vi "Day 5.2 - overlap with diagnals.vi"(11 "input":string[](array[string])) -> (3 "output":u32)   [LabVIEW 2021]
uses:
  Controls/Thermal position.ctl
  Controls/vent position.ctl
panel:
  out "Intensity Graph":i32[][](graph)
  out "vents":i32[][](array[numeric])
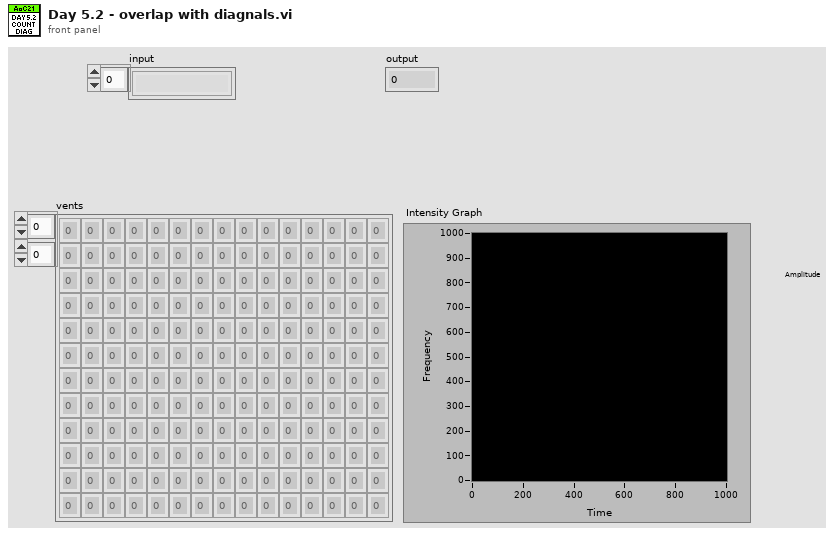
[diagram p1: front panel]
types:
  T1 = typedef "Thermal position.ctl" = cluster{"Start Vent position":T2, "End Vent position":T2}
  T2 = typedef "vent position.ctl" = cluster{"x":i32, "y":i32}
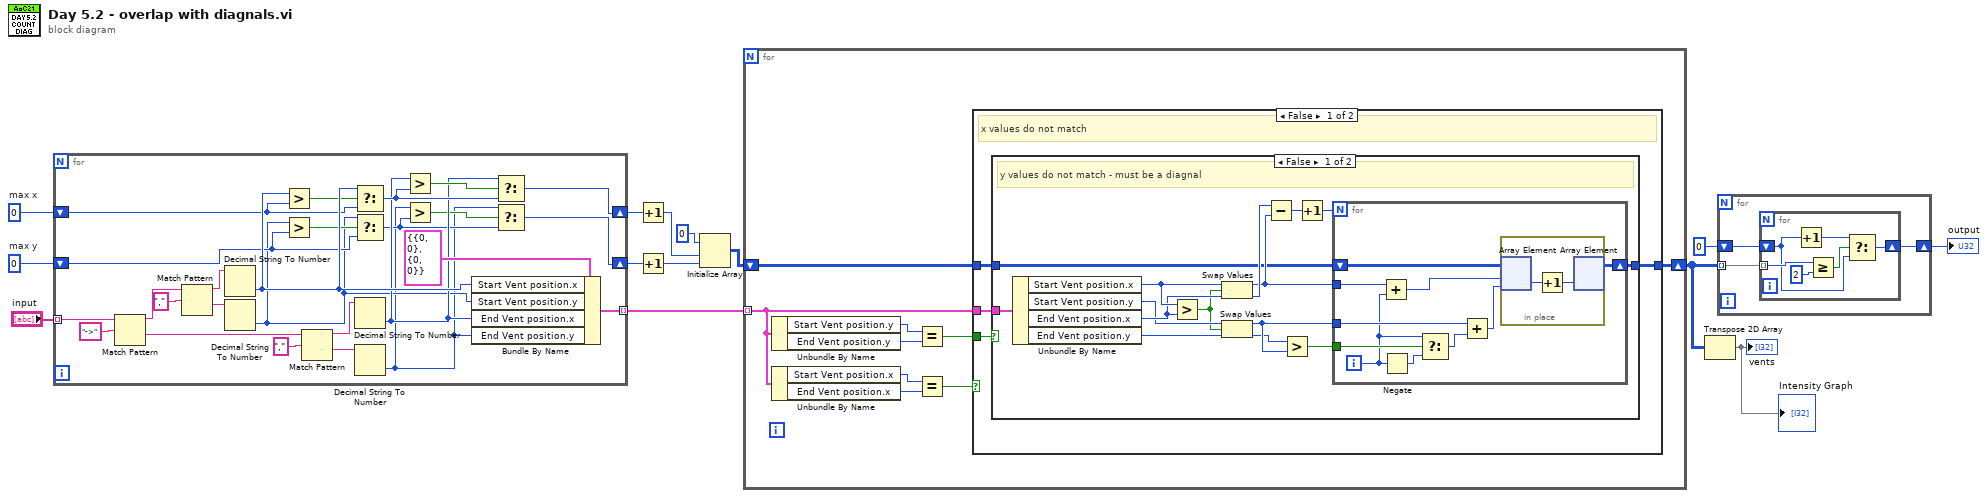
[diagram p0: block diagram]
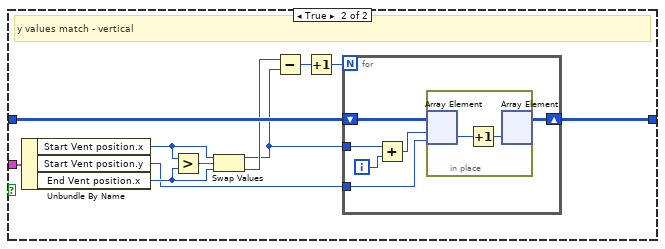
[diagram p2: hidden frame]
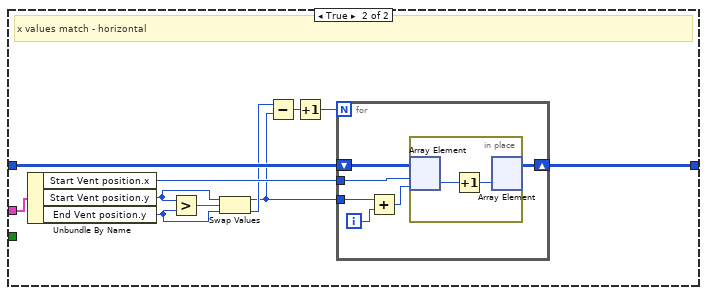
[diagram p3: hidden frame]
diagram:
  w11 = 0  # max y
  w12 = 0  # max x
  n1 = for {
    tunnel: "input" -> [w40] mode=indexing
    tunnel: [w29] -> w13 mode=indexing
    shift-right: [w24] -> w9
    shift-left: w12 -> [w26]
    shift-right: [w18] -> w8
    shift-left: w11 -> [w17]
    n2 = Match Pattern(string=w40, regular expression="->") -> (before substring=w38:string, after substring=w35:string)  [unwired: 1 in, 2 out]
    n3 = Match Pattern(string=w38, regular expression=",") -> (before substring=w32:string, after substring=w31:string)  [unwired: 1 in, 2 out]
    n4 = Decimal String To Number(string=w32) -> (number=w28:i32)  [unwired: 2 in, 1 out]
    n5 = Decimal String To Number(string=w31) -> (number=w16:i32)  [unwired: 2 in, 1 out]
    n6 = Greater?(x=w28, y=w26) -> (0:w27:bool)
    n7 = Greater?(x=w16, y=w17) -> (0:w21:bool)
    n8 = Match Pattern(string=w35, regular expression=",") -> (before substring=w34:string, after substring=w33:string)  [unwired: 1 in, 2 out]
    n9 = Select(t=w28, s=w27, f=w26) -> (s? t:f=w23:i32)
    n10 = Select(t=w16, s=w21, f=w17) -> (s? t:f=w19:i32)
    n11 = Decimal String To Number(string=w34) -> (number=w22:i32)  [unwired: 2 in, 1 out]
    n12 = Decimal String To Number(string=w33) -> (number=w15:i32)  [unwired: 2 in, 1 out]
    n13 = Greater?(x=w22, y=w23) -> (0:w25:bool)
    n14 = Greater?(x=w15, y=w19) -> (0:w20:bool)
    n15 = Bundle By Name(cluster=T1 {"Start Vent position"={"x"=0, "y"=0}, "End Vent position"={"x"=0, "y"=0}} ("Hydrothermal"), "Start Vent position.x"=w28, "Start Vent position.y"=w16, "End Vent position.x"=w22, "End Vent position.y"=w15) -> (w29:T1)
    n16 = Select(t=w22, s=w25, f=w23) -> (s? t:f=w24:i32)
    n17 = Select(t=w15, s=w20, f=w19) -> (s? t:f=w18:i32)
  }
  n18 = Increment(x=w9) -> (x+1=w6:i32)
  n19 = Increment(x=w8) -> (x+1=w5:i32)
  n20 = Initialize Array(0, w6, w5) -> (w7:i32[][])
  n21 = for {
    tunnel: w13 -> [w42] mode=indexing
    shift-right: [w41] -> w2
    shift-left: w7 -> [w44]
    n22 = Unbundle By Name(w42) -> ("Start Vent position.y"=w49:i32, "End Vent position.y"=w48:i32)
    n23 = Unbundle By Name(w42) -> ("Start Vent position.x"=w46:i32, "End Vent position.x"=w45:i32)
    n24 = Equal?(x=w49, y=w48) -> (x = y?=w43:bool)
    n25 = Equal?(x=w46, y=w45) -> (x = y?=w47:bool)
    n26 = case shown="False" w47 {
      tunnel: w44 -> [w51 w110]
      tunnel: [w50 w104] -> w41
      tunnel: w43 -> [w53 _]
      tunnel: w42 -> [w52 w101]
      frame False {
        # "x values do not match"
        n27 = case shown="False" w53 {
          tunnel: [w61 w88] -> w50
          tunnel: w52 -> [w60 w91]
          tunnel: w51 -> [w62 w87]
          frame False {
            # "y values do not match - must be a diagnal"
            n28 = Unbundle By Name(w60) -> ("Start Vent position.x"=w65:i32, "Start Vent position.y"=w59:i32, "End Vent position.x"=w64:i32, "End Vent position.y"=w58:i32)
            n29 = Greater?(x=w65, y=w64) -> (0:w57:bool)
            n30 = Swap Values(12:w65, 13:w57, 14:w64) -> (1:w66:i32, 3:w67:i32)
            n31 = Swap Values(12:w59, 13:w57, 14:w58) -> (1:w55:i32, 3:w54:i32)
            n32 = Subtract(x=w67, y=w66) -> (x-y=w68:i32)
            n33 = Greater?(x=w54, y=w55) -> (0:w56:bool)
            n34 = Increment(x=w68) -> (x+1=w63:i32)
            n35 = for {
              N: w63 -> [_]
              tunnel: w66 -> [w78]
              shift-right: [w75] -> w61
              shift-left: w62 -> [w77]
              tunnel: w55 -> [w74]
              tunnel: w56 -> [w72]
              i -> [w69]
              n36 = Add(x=w78, y=w69) -> (x+y=w76:i32)
              n37 = Negate(x=w69) -> (-x=w71:i32)
              n38 = Select(t=w69, s=w72, f=w71) -> (s? t:f=w70:i32)
              n39 = Add(x=w74, y=w70) -> (x+y=w73:i32)
              n40 = in-place {
                n41 = in-place-array #1(w77, w76, w73) -> (w80:i32)
                n42 = Increment(x=w80) -> (x+1=w79:i32)
                n43 = in-place-array #1(w79) -> (w75:i32[][])  [unwired: 2 out]
              }
            }
          }
          frame True {
            # "y values match - vertical"
            n44 = Unbundle By Name(w91) -> ("Start Vent position.x"=w84:i32, "Start Vent position.y"=w82:i32, "End Vent position.x"=w83:i32)
            n45 = Greater?(x=w84, y=w83) -> (0:w90:bool)
            n46 = Swap Values(12:w84, 13:w90, 14:w83) -> (1:w85:i32, 3:w86:i32)
            n47 = Subtract(x=w86, y=w85) -> (x-y=w89:i32)
            n48 = Increment(x=w89) -> (x+1=w81:i32)
            n49 = for {
              N: w81 -> [_]
              tunnel: w82 -> [w93]
              tunnel: w85 -> [w96]
              shift-right: [w92] -> w88
              shift-left: w87 -> [w95]
              i -> [w97]
              n50 = Add(x=w96, y=w97) -> (x+y=w94:i32)
              n51 = in-place {
                n52 = in-place-array #2(w95, w94, w93) -> (w99:i32)
                n53 = Increment(x=w99) -> (x+1=w98:i32)
                n54 = in-place-array #2(w98) -> (w92:i32[][])  [unwired: 2 out]
              }
            }
          }
        }
      }
      frame True {
        # "x values match - horizontal"
        n55 = Unbundle By Name(w101) -> ("Start Vent position.x"=w109:i32, "Start Vent position.y"=w100:i32, "End Vent position.y"=w107:i32)
        n56 = Greater?(x=w100, y=w107) -> (0:w108:bool)
        n57 = Swap Values(12:w100, 13:w108, 14:w107) -> (1:w103:i32, 3:w105:i32)
        n58 = Subtract(x=w105, y=w103) -> (x-y=w106:i32)
        n59 = Increment(x=w106) -> (x+1=w102:i32)
        n60 = for {
          N: w102 -> [_]
          tunnel: w109 -> [w115]
          tunnel: w103 -> [w113]
          shift-right: [w111] -> w104
          shift-left: w110 -> [w116]
          i -> [w114]
          n61 = Add(x=w113, y=w114) -> (x+y=w112:i32)
          n62 = in-place {
            n63 = in-place-array #3(w116, w115, w112) -> (w118:i32)
            n64 = Increment(x=w118) -> (x+1=w117:i32)
            n65 = in-place-array #3(w117) -> (w111:i32[][])  [unwired: 2 out]
          }
        }
      }
    }
  }
  n66 = Transpose 2D Array(2D array=w2) -> (transposed array=→"vents" →"Intensity Graph":i32[][])
  n67 = for {
    tunnel: w2 -> [w121] mode=indexing
    shift-right: [w119] -> w3
    shift-left: 0 -> [w120]
    n68 = for {
      tunnel: w121 -> [w127] mode=indexing
      shift-right: [w122] -> w119
      shift-left: w120 -> [w124]
      n69 = Increment(x=w124) -> (x+1=w123:i32)
      n70 = Greater Or Equal?(x=w127, y=2) -> (x >= y?=w125:bool)
      n71 = Select(t=w123, s=w125, f=w124) -> (s? t:f=w122:i32)
    }
  }
  "output" <- w3
